vi "LWXPS_CPUTemperatureAndFanSpeedGet.vi"(0 "XPS Reference IN":refnum<k24>, 5 "LabVIEW error IN":errorcluster) -> (14 "XPS Reference OUT":refnum<k24>, 15 "Returned error code":i32, 16 "CPU Temperature":dbl, 17 "CPU Fan Speed":dbl, 18 "XPS Error String":string, 19 "LabVIEW error OUT":errorcluster)   [LabVIEW 2014]
uses:
  D:/XPSQ8_LabView_Library/Development/Source/Dll/Newport.XPS.CommandInterface.dll
  Dll/Newport.XPS.CommandInterface.dll
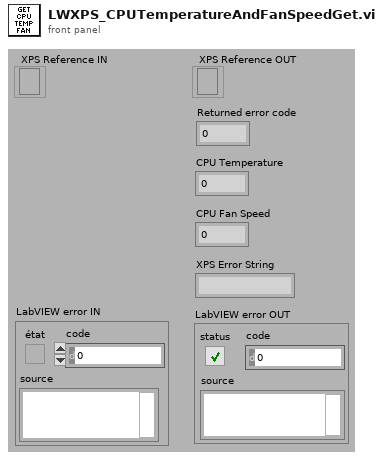
[diagram p1: front panel]
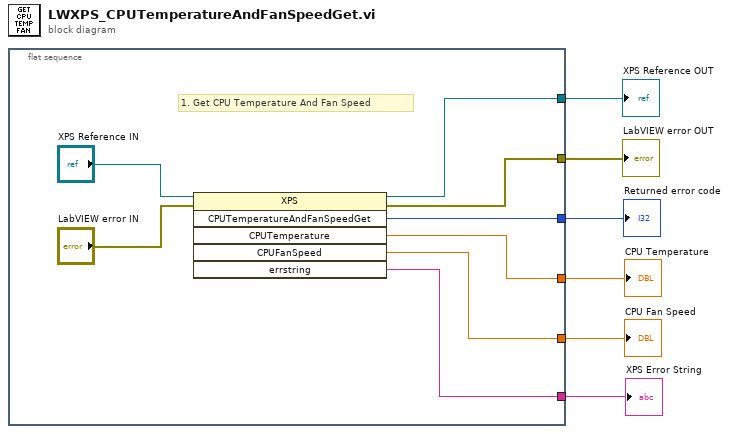
[diagram p0: block diagram]
diagram:
  n1 = flat-sequence {
    tunnel: [w10] -> w6
    tunnel: [w14] -> w5
    tunnel: [w11] -> w4
    tunnel: [w7] -> w2
    tunnel: [w8] -> w3
    tunnel: [w9] -> w1
    frame #0 {
      # "1. Get CPU Temperature And Fan Speed"
      n2 = invoke class="XPS" method="CPUTemperatureAndFanSpeedGet"(reference="XPS Reference IN", error in="LabVIEW error IN") -> (reference out=w10:refnum<k24>, error out=w14:errorcluster, "CPUTemperatureAndFanSpeedGet"=w11:i32, "CPUTemperature"=w8:dbl, "CPUFanSpeed"=w7:dbl, "errstring"=w9:string)  [unwired: 4 in]
    }
  }
  "XPS Reference OUT" <- w6
  "LabVIEW error OUT" <- w5
  "Returned error code" <- w4
  "CPU Temperature" <- w3
  "CPU Fan Speed" <- w2
  "XPS Error String" <- w1
